vi "remove tag select.vi"(8 "error in":errorcluster, 10 "tag select":string, 11 "object ref in":T1) -> (0 "error out":errorcluster)   [LabVIEW 2013, in "tag select module editor node.lvclass"]
uses:
  tag select module editor node.lvclass
  object ref.ctl
  <vilib>/NI/Tag Bus Data Framework/Configuration Editor/Classes/Engine Parent/Engine Parent Editor Node.lvclass
  tag select module editor node.lvclass/tag select module editor node.ctl
  <vilib>/NI/Configuration Framework/serializable configuration/NISE_CEF_serializable configuration.lvclass/NISE_CEF_serializable configuration.ctl
  <vilib>/Utility/LVClass/Get LV Class Name.vi
  <vilib>/NI/Configuration Framework/error generator/NISE_error generator.vi
  <vilib>/NI/Configuration Framework/serializable configuration/NISE_CEF_serializable configuration.lvclass
  <vilib>/NI/Module Execution Interface/Engine Configuration/engine configuration.lvclass
  module/configuration/tag select module configuration.lvclass
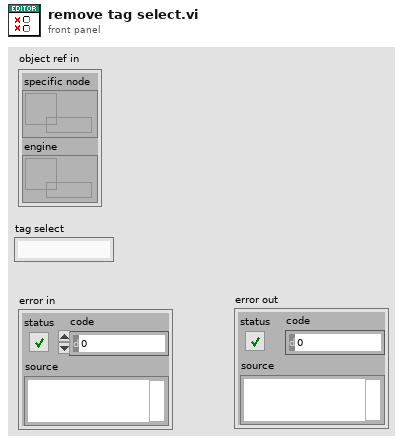
[diagram p1: front panel]
types:
  T1 = typedef "tag select module editor node.lvclass/object ref.ctl" = cluster{"specific node":refnum<data-value>, "engine":refnum<data-value>}
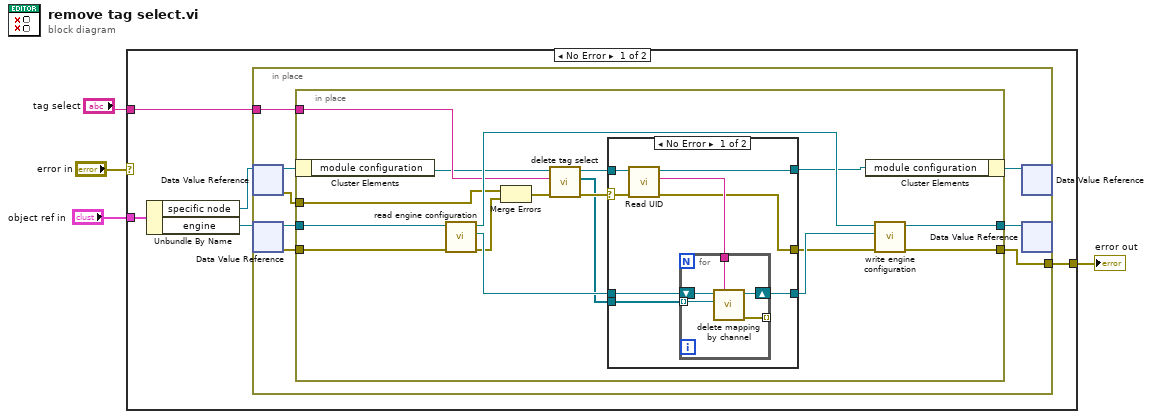
[diagram p0: block diagram]
diagram:
  n1 = case shown="No Error" "error in" {
    selector: "error in" -> [_ w51]
    tunnel: [w9 w51] -> w4
    tunnel: "object ref in" -> [w6 _]
    tunnel: "tag select" -> [w5 _]
    frame No Error {
      n2 = Unbundle By Name(w6) -> ("specific node"=w7:refnum<data-value>, "engine"=w8:refnum<data-value>)
      n3 = in-place {
        in-place-border: [w16] -> w9
        in-place-border: w5 -> [w12]
        n4 = in-place-dvr #1(w7) -> (w11:refnum<class "tag select module editor node.lvclass">, w13:errorcluster)
        n5 = in-place-dvr #2(w8) -> (w15:refnum<class "Engine Parent Editor Node.lvclass">, w14:errorcluster)
        n6 = in-place {
          in-place-border: [w34] -> w17
          in-place-border: [w33] -> w16
          in-place-border: w15 -> [w31]
          in-place-border: w14 -> [w30]
          in-place-border: w13 -> [w26]
          in-place-border: w12 -> [w21]
          n7 = in-place-cluster #3(w11) -> ("module configuration"=w19:refnum<class "tag select module configuration.lvclass">)
          n8 = call <vilib>:"read engine configuration.vi"("error in"=w30, "Engine Parent Editor Node in"=w31) -> ("error out"=w27:errorcluster, "engine configuration"=w29:refnum<class "engine configuration.lvclass">, "Engine Parent Editor Node out"=w28:refnum<class "Engine Parent Editor Node.lvclass">)  [unwired: 7 in]
          n9 = Merge Errors(w26, w27) -> (w25:errorcluster)
          n10 = call "delete tag select.vi"("error in"=w25, "tag selecct name"=w21, "tag select module configuration in"=w19) -> ("error out"=w24:errorcluster, "deleted channels"=w23:refnum<class "TBM channel.lvclass">[], "tag select module configuration out"=w20:refnum<class "tag select module configuration.lvclass">)  [unwired: 6 in]
          n11 = case shown="No Error" w24 {
            selector: w24 -> [w38 w49]
            tunnel: [w37 w49] -> w22
            tunnel: w20 -> [w40 w48]
            tunnel: w29 -> [w42 w50]
            tunnel: [w41 w50] -> w32
            tunnel: w23 -> [w36 _]
            tunnel: [w35 w48] -> w18
            frame No Error {
              n12 = call <vilib>:"Read UID.vi"("error in"=w38, "configuration in"=w40) -> ("error out"=w37:errorcluster, "instance id"=w39:string, "configuration out"=w35:refnum<class "tag select module configuration.lvclass">)  [unwired: 7 in]
              n13 = for {
                tunnel: w39 -> [w45]
                shift-right: [w46] -> w41
                shift-left: w42 -> [w47]
                tunnel: [w44] -> _ mode=indexing
                tunnel: w36 -> [w43] mode=indexing
                n14 = call <vilib>:"delete mapping by channel.vi"("owner ID"=w45, "channel"=w43, "engine configuration in"=w47) -> ("error out"=w44:errorcluster, "engine configuration out"=w46:refnum<class "engine configuration.lvclass">)  [unwired: 7 in]
              }
            }
            frame Error {
            }
          }
          n15 = in-place-cluster #3("module configuration"=w18) -> (w10:refnum<class "tag select module editor node.lvclass">)
          n16 = call <vilib>:"write engine configuration.vi"("error in"=w22, "engine configuration"=w32, "Engine Parent Editor Node in"=w28) -> ("error out"=w33:errorcluster, "Engine Parent Editor Node out"=w34:refnum<class "Engine Parent Editor Node.lvclass">)  [unwired: 7 in]
        }
        n17 = in-place-dvr #1(w10) -> ()  [unwired: 2 out]
        n18 = in-place-dvr #2(w17) -> ()  [unwired: 2 out]
      }
    }
    frame Error {
    }
  }
  "error out" <- w4
